vi "Add.vi"(6 "Options":T1={"DbType"=-1, "Direction"=-1, "Size"=-1, "Precision"=255, "Scale"=255} {"Direction" items=["Input"=1, "Output"=2, "InputOutput"=3, "ReturnValue"=6]; "DbType" items=["AnsiString"=0, "Binary"=1, "Byte"=2, "Boolean"=3, "Currency"=4, "Date"=5, "DateTime"=6, "Decimal"=7, "Double"=8, "Guid"=9, "Int16"=10, "Int32"=11, "Int64"=12, "Object"=13, "SByte"=14, "Single"=15, "String"=16, "Time"=17, "UInt16"=18, "UInt32"=19, "UInt64"=20, "VarNumeric"=21, "AnsiStringFixedLength"=22, "StringFixedLength"=23, "Xml"=25, "DateTime2"=26, "DateTimeOffset"=27]}, 8 "error in (no error)":errorcluster, 9 "value":variant, 10 "name":string, 11 "ADOParameter in":refnum<class "ADOParameter.lvclass">) -> (0 "error out":errorcluster, 3 "ADOParameter out":refnum<class "ADOParameter.lvclass">)   [LabVIEW 2020, in "ORM_ADONet.lvlib" / "ADOParameter.lvclass"]
uses:
  ADOParameter.lvclass
  <vilib>/Viviota/shared/ORM.lvlibp/ORM/DynamicParameters/DynamicParameters.lvclass
  C:/Program Files/National Instruments/LabVIEW 2020/vi.lib/Viviota/shared/ORM.lvlibp/ORM/DynamicParameters/DynamicParameters.lvclass
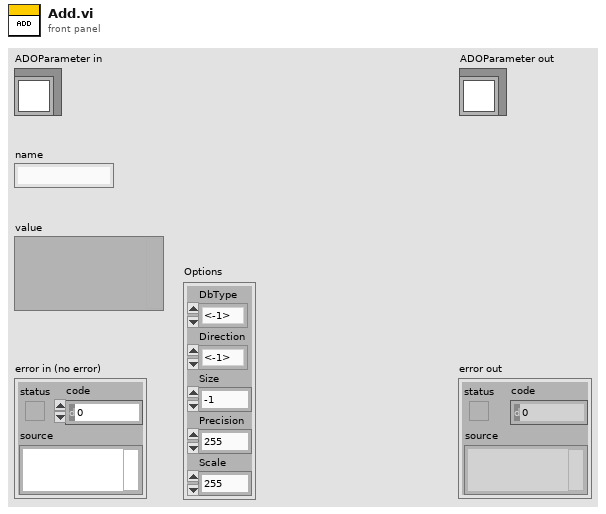
[diagram p1: front panel]
types:
  T1 = cluster{"DbType":i32, "Direction":i32, "Size":i32, "Precision":u8, "Scale":u8}
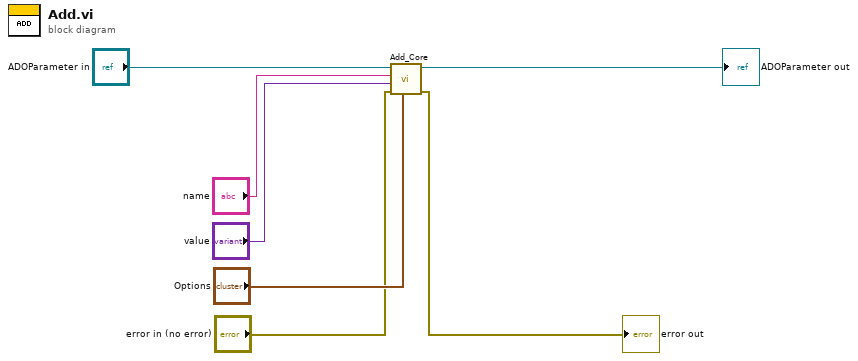
[diagram p0: block diagram]
diagram:
  n1 = call <vilib>:"Add_Core.vi"("Options"="Options", "error in (no error)"="error in (no error)", "value"="value", "name"="name", "DynamicParameters in"="ADOParameter in") -> ("error out"=→"error out":errorcluster, "DynamicParameters out"=→"ADOParameter out":refnum<class "ADOParameter.lvclass">)  [unwired: 5 in]
